vi "select_device.vi"(8 "error in (no error)":errorcluster, 10 "device (1)":i32=1, 11 "Handle in":i64) -> (0 "error out":errorcluster, 2 "Return (<0 is error)":i32, 3 "Handle out":i64)   [LabVIEW 2016, in "OSB_uMp_library.lvlib"]
doc: "Once connected to a hub/controller, this VI selects a uMp. This is required before calling functions that don't have an argument for selecting uMp, as they will attempt to use the selection made through this VI."
uses:
  OSB_uMp_library.lvlib
  ump.dll
panel:
  # "By Stuart Box at OxSyBio Ltd, 2017\n\nThis software is provided WITHOUT ANY WARRANTY; without even the implied warranty of MERCHANTABILITY or FITNESS FOR A PARTICULAR PURPOSE.\n\ninfo@oxsybio.com\n\nOxSyBio Ltd, The Walbrook Building, 25 Walbrook, London, EC4N 8AF"
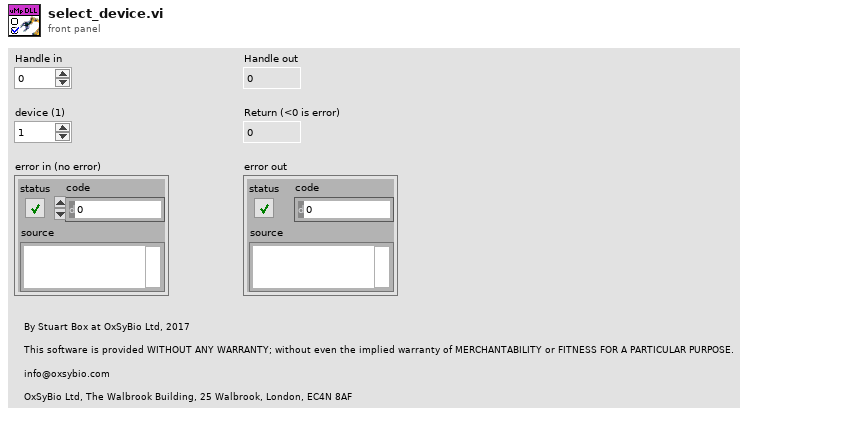
[diagram p1: front panel]
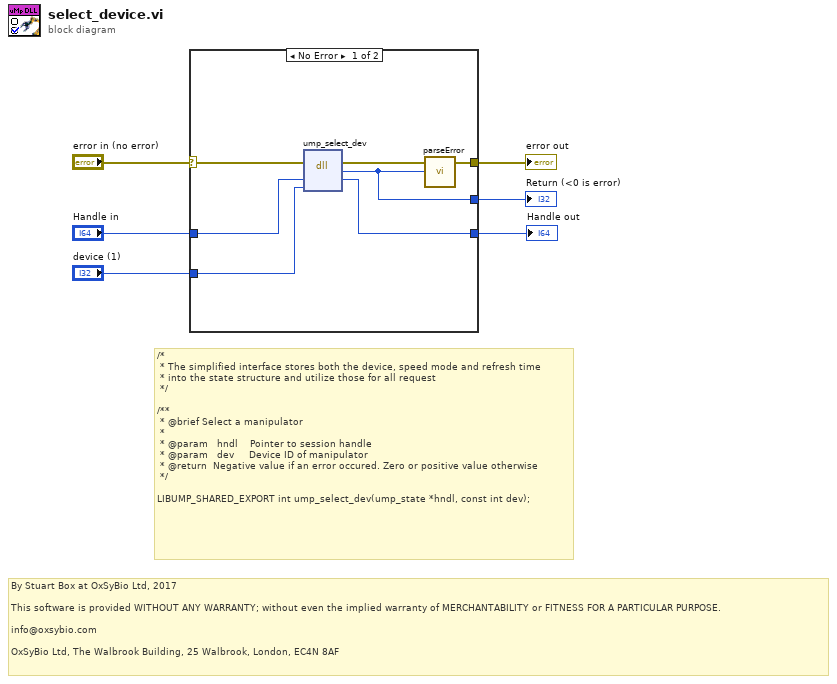
[diagram p0: block diagram]
diagram:
  # "By Stuart Box at OxSyBio Ltd, 2017\n\nThis software is provided WITHOUT ANY WARRANTY; without even the implied warranty of MERCHANTABILITY or FITNESS FOR A PARTICULAR PURPOSE.\n\ninfo@oxsybio.com\n\nOxSyBio Ltd, The Walbrook Building, 25 Walbrook, London, EC4N 8AF"
  # "/*\n * The simplified interface stores both the device, speed mode and refresh time\n * into the state structure and utilize those for all request\n */\n\n/**\n * @brief Select a manipulator\n *\n * @param   hndl    Pointer to session handle\n * @param   dev     Device ID of manipulator\n * @return  Negative value if an error occured. Zero or positive value otherwise\n */\n\nLIBUMP_SHARED_EXPORT int ump_select_dev(ump_state *hndl, const int dev);"
  n1 = case shown="No Error" "error in (no error)" {
    selector: "error in (no error)" -> [w10 w15]
    tunnel: "Handle in" -> [w13 w14]
    tunnel: [w8 w15] -> w5
    tunnel: "device (1)" -> [w12 _]
    tunnel: [w7 _] -> w3
    tunnel: [w11 w14] -> w2
    frame No Error {
      n2 = dll-call lib="C:/Users/Stu/Desktop/OSB LabVIEW uMp/uMp_library/ump.dll" fn="ump_select_dev"(error in=w10, "handle"=w13, "device"=w12) -> (error out=w9:errorcluster, "return"=w7:i32, "handle"=w11:i64)  [unwired: 3 in, 1 out]
      n3 = call "parseError.vi"("Error In"=w9, "ump dll return value (<0 is error)"=w7) -> ("Error Out"=w8:errorcluster)  [unwired: 24 in, 1 out]
    }
    frame Error {
    }
  }
  "error out" <- w5
  "Return (<0 is error)" <- w3
  "Handle out" <- w2
